vi "Main - ZMQ.vi"(8 "error in (no error)":T1) -> (0 "error out":T1)   [LabVIEW 2019, in "Communication Interface.lvlib"]
uses:
  Communication Interface.lvlib
  Intertarget communication/Status + response + data cluster.ctl
  module state.ctl
  module data.ctl
  Intertarget communication/CR_master_class/CR_master.lvclass
  Intertarget communication/CR slave_class/CR slave.lvclass
  5bf6cc24-2521-4779-a80f-885c0f377251.vi
  ZMQ_mmWave_class/ZMQ_mmWave.lvclass
  C:/Barkhausen mmWave radar/Development/modules/mmw_instrument/src_LabVIEW/Host/Intertarget communication/CR slave_class/CR slave.lvclass
  Intertarget communication/UE_master_class/UE_master.lvclass
  C:/Barkhausen mmWave radar/Development/modules/mmw_instrument/src_LabVIEW/Host/Intertarget communication/CR_master_class/CR_master.lvclass
  SubVIs/Shared/Comm GV.vi
  SubVIs/Shared/System GV.vi
  Intertarget communication/CommandResponse communication.lvlib
  SubVIs/Shared/Shared.lvlib
  Intertarget communication/NS slave_class/NS slave.lvclass
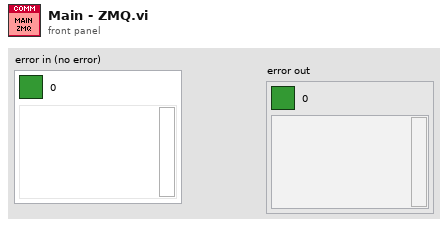
[diagram p1: front panel]
types:
  T1 = cluster{"Boolean Round":bool, "code":i32, "source":string}
  T2 = typedef "Communication Interface.lvlib/module state.ctl" = enum16{"init", "wait on connection", "communication", "close"}
  T3 = typedef "CommandResponse communication.lvlib/Status + response + data cluster.ctl" = cluster{"message":string, "response":string, "data":variant}
  T4 = typedef "Communication Interface.lvlib/module data.ctl" = cluster{"dummy":dbl, "HW Control":refnum<class "CR_master.lvclass">, "Command interface":refnum<class "CR slave.lvclass">}
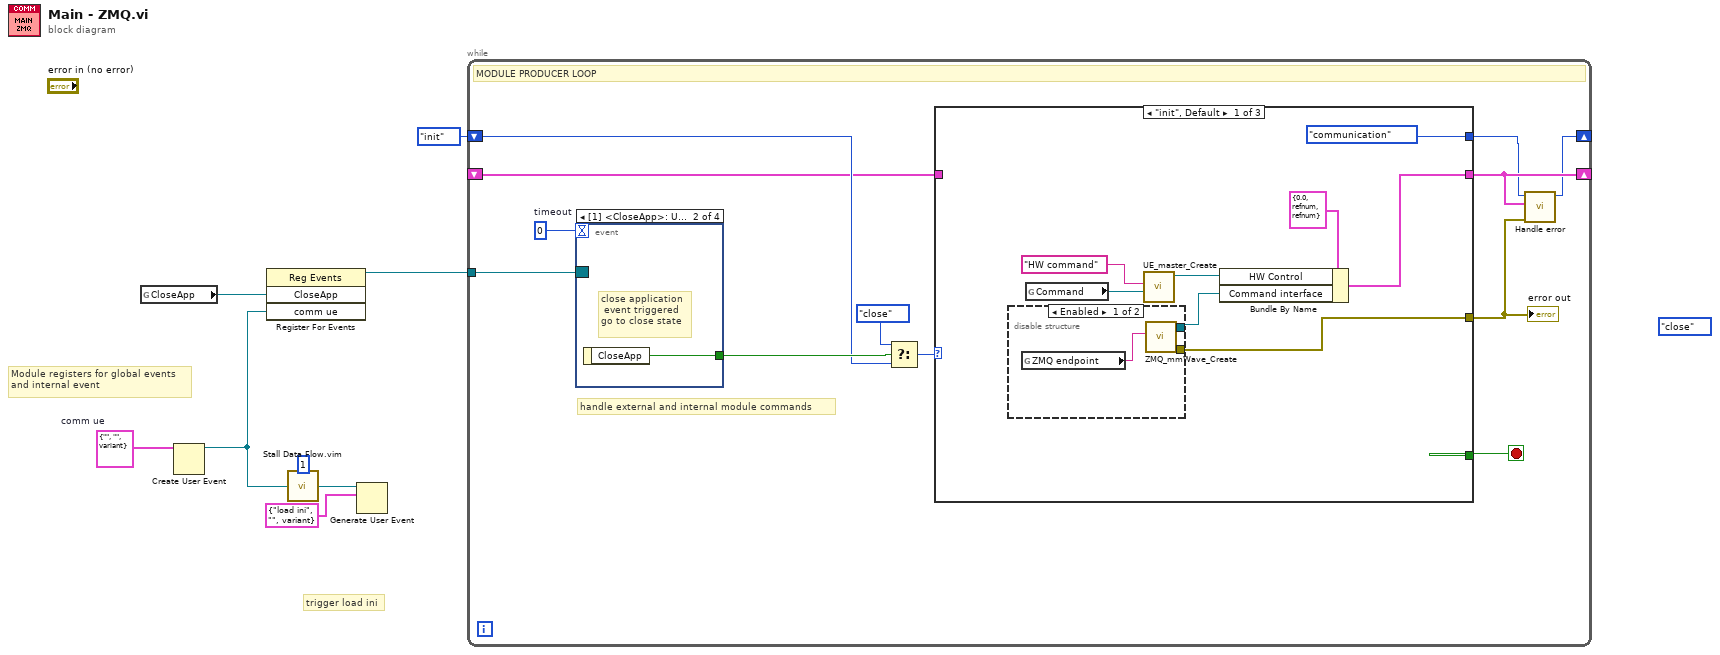
[diagram p0: block diagram]
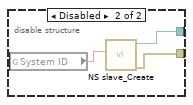
[diagram p2: hidden frame]
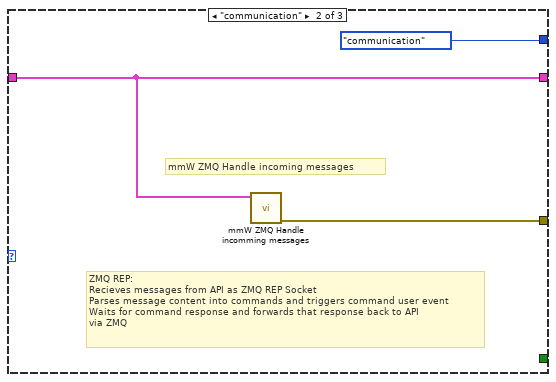
[diagram p3: hidden frame]
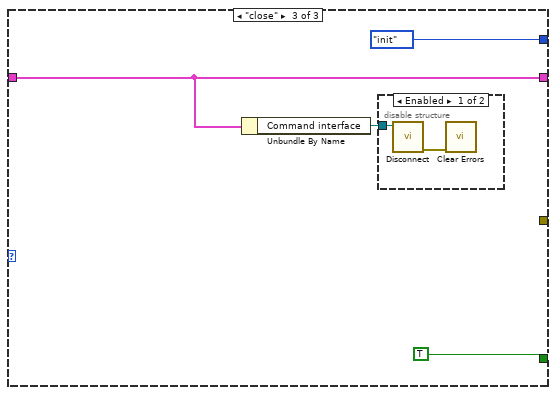
[diagram p4: hidden frame]
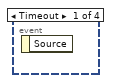
[diagram p6: hidden frame]
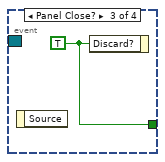
[diagram p7: hidden frame]
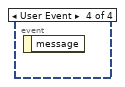
[diagram p8: hidden frame]
diagram:
  w4 = T3 {"message"="", "response"="", "data"=variant}  # comm ue
  (unwired) module_state."close" ("module states")
  # "trigger load ini"
  # "Module registers for global events\nand internal event"
  n1 = global read "Comm GV.vi" "CloseApp"() -> (w2:refnum<user-event>)
  n2 = Create User Event(user event datatype=w4) -> (user event=w7:refnum<user-event>)  [unwired: 1 in, 1 out]
  n3 = register-events(w2, w7) -> (reference out=w8:refnum<event-registration>)  [unwired: 2 in, 1 out]
  n4 = call "Stall Data Flow.vim"("value in"=w7, "milliseconds to wait"=u32 1) -> ("value out"=w6:refnum<user-event>)  [unwired: 1 out]
  n5 = Generate User Event(user event=w6, event data cluster=T3 {"message"="load ini", "response"="", "data"=variant} ("internal command")) -> ()  [unwired: 2 in, 2 out]
  n6 = while {
    tunnel: w8 -> [w20]
    shift-right: [w13] -> _
    shift-left: _ -> [w14]
    shift-right: [w9] -> _
    shift-left: module_state."init" ("module states") -> [w17]
    stop <- w12 stop-if-true
    w19 = 0  # timeout
    # "handle external and internal module commands"
    # "MODULE PRODUCER LOOP"
    n7 = event shown="[1] <CloseApp>: User Event" {
      selector: w20 -> [_ _ _ _]
      dyn-events: _ -> [_ _ _ _]
      timeout: w19 -> [_ _ _ _]
      tunnel: [_ w44 w45 _] -> w18
      event Timeout {
        n8 = event-data() -> ()  [unwired: 1 in, 1 out]
      }
      event User Event {
        # "close application\n event triggered\ngo to close state"
        n9 = event-data() -> ("CloseApp"=w44:bool)  [unwired: 1 in]
      }
      event Panel Close? {
        w45 = TRUE ("Discard?")
        n10 = event-data() -> ()  [unwired: 1 in, 1 out]
        n11 = event-data("Discard?"=w45) -> ()  [unwired: 1 in, 1 out]
      }
      event User Event {
        n12 = event-data() -> ()  [unwired: 1 in, 1 out]
      }
    }
    n13 = Select(t=module_state."close", s=w18, f=w17) -> (s? t:f=w15:T2)
    n14 = case shown="\"init\", Default" w15 {
      tunnel: [module_state."communication" ("module states") module_state."communication" ("t") module_state."init" ("t")] -> w10
      tunnel: [w22 w37 w40] -> w13
      tunnel: w14 -> [_ w37 w40]
      tunnel: [_ _ TRUE] -> w12
      tunnel: [w21 w36 _] -> w11
      frame "init", Default {
        n15 = disable-structure shown="Enabled" {
          disable-tunnel: [w31 w33] -> w27
          disable-tunnel: [w30 w32] -> w21
          frame Enabled {
            n16 = global read "System GV.vi" "ZMQ endpoint"() -> (w29:string)
            n17 = call "ZMQ_mmWave_Create.vi"("endpoint"=w29) -> ("error out"=w30:errorcluster, "reference out"=w31:refnum<class "ZMQ_mmWave.lvclass">)  [unwired: 9 in]
          }
          frame Disabled {
            n18 = global read "System GV.vi" "System ID"() -> (w34:string)
            n19 = call "NS slave_Create.vi"("ID"=w34) -> ("error out"=w32:errorcluster, "reference out"=w33:refnum<class "NS slave.lvclass">)  [unwired: 9 in]
          }
        }
        n20 = global read "Comm GV.vi" "Command"() -> (w24:refnum<user-event>)
        n21 = call "UE_master_Create.vi"("Command UE"=w24, "ID"="HW command") -> ("reference out"=w26:refnum<class "UE_master.lvclass">)  [unwired: 8 in, 1 out]
        n22 = Bundle By Name(cluster=T4 {"dummy"=0.0, "HW Control"=refnum, "Command interface"=refnum} ("module loopdata"), "HW Control"=w26, "Command interface"=w27) -> (w22:T4)
      }
      frame "communication" {
        # "mmW ZMQ Handle incoming messages"
        # "ZMQ REP:\nRecieves messages from API as ZMQ REP Socket\nParses message content into commands and triggers command user event\nWaits for command response and forwards that response back to API\nvia ZMQ"
        n23 = call "mmW ZMQ Handle incomming messages.vi"("module loopdata"=w37) -> ("error out"=w36:errorcluster)  [unwired: 9 in, 1 out]
      }
      frame "close" {
        n24 = Unbundle By Name(w40) -> ("Command interface"=w39:refnum<class "CR slave.lvclass">)
        n25 = disable-structure shown="Enabled" {
          disable-tunnel: w39 -> [w43 _]
          frame Enabled {
            n26 = call-dynamic "Disconnect.vi"("reference in"=w43) -> ("error out"=w42:errorcluster)  [unwired: 9 in, 1 out]
            n27 = call <vilib>:"Clear Errors.vi"("error in (no error)"=w42) -> ()  [unwired: 5 in, 2 out]
          }
          frame Disabled {
          }
        }
      }
    }
    "error out" <- w11
    n28 = call "Handle error.vi"("error in (no error)"=w11, "module loopdata"=w13, "state in"=w10) -> ("state out"=w9:T2)  [unwired: 8 in]
  }
